vi "links weiter.vi"(8 "error in (no error)":errorcluster caption="Fehler (Eingang, kein Fehler)", 11 "Device ID":T1(ring)) -> (0 "error out":errorcluster caption="Fehler (Ausgang)", 2 "geradeaus?":bool, 3 "Device ID Out":T1(ring))   [LabVIEW 2010]
uses:
  globale Variable 1.vi
panel:
  out "aktuelle Position":i32
  in  "pneumatik?":bool
  in  "ende?":bool
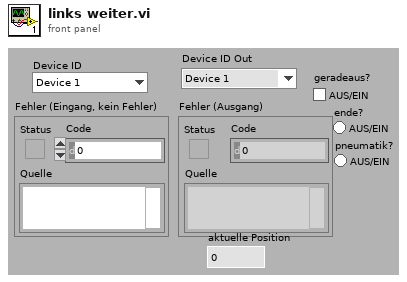
[diagram p1: front panel]
types:
  T1 = enum16{"Device 1", "Device 2", "Device 3", "Device 4", "Device 5", "Device 6", "Device 7", "Device 8"}
  T2 = enum8{"Output 1 (O1)", "Output 2 (O2)", "Output 3 (O3)", "Output 4 (O4)", "Output 5 (O5)", "Output 6 (O6)", "Output 7 (O7)", "Output 8 (O8)"}
  T3 = enum8{"Robo Interface", "Extension 1", "Extension 2", "Extension 3"}
  T4 = enum8{"Power 1", "Power 2", "Power 3", "Power 4", "Power 5", "Power 6", "Power 7", "Power 8"}
  T5 = enum8{"Input 1 (I1)", "Input 2 (I2)", "Input 3 (I3)", "Input 4 (I4)", "Input 5 (I5)", "Input 6 (I6)", "Input 7 (I7)", "Input 8 (I8)"}
  T6 = enum8{"Goes High", "Goes Low", "Goes High or Low"}
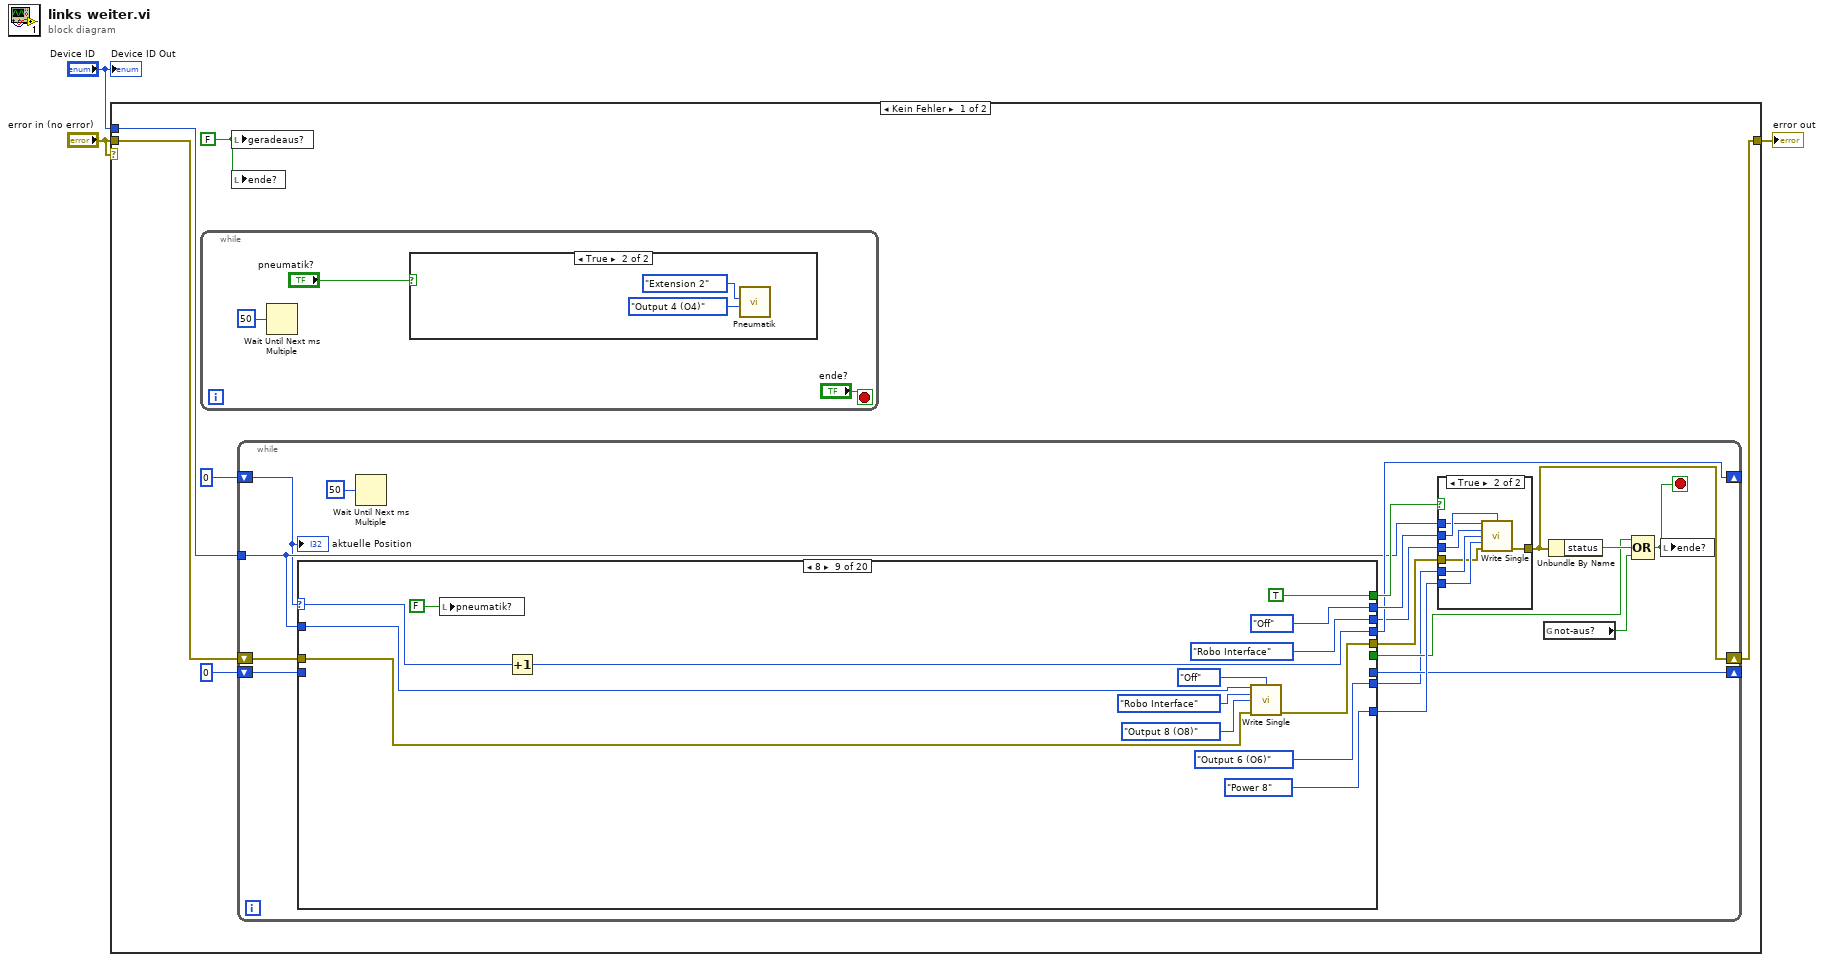
[diagram p0: block diagram]
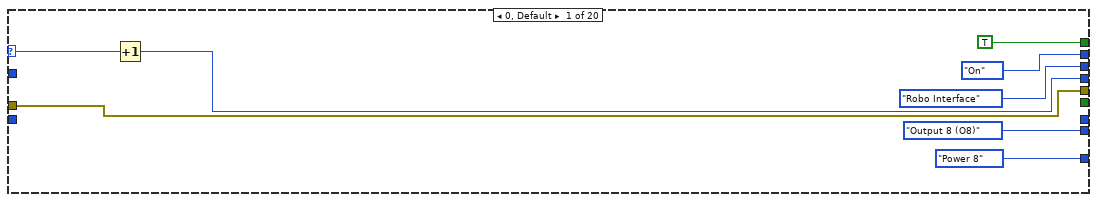
[diagram p3: hidden frame]
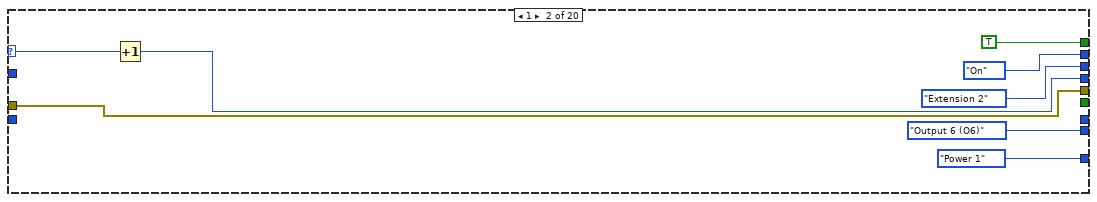
[diagram p4: hidden frame]
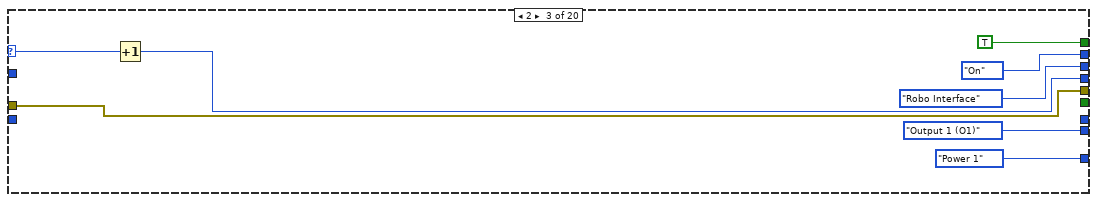
[diagram p5: hidden frame]
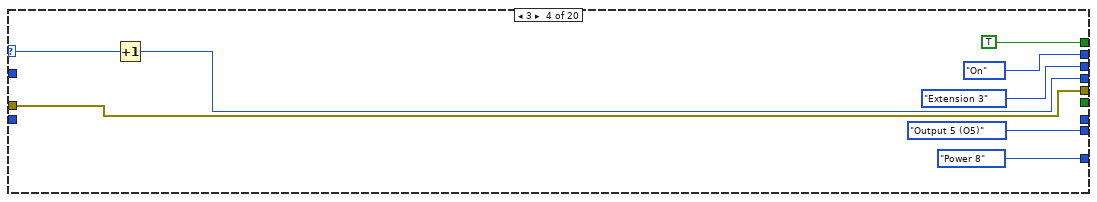
[diagram p6: hidden frame]
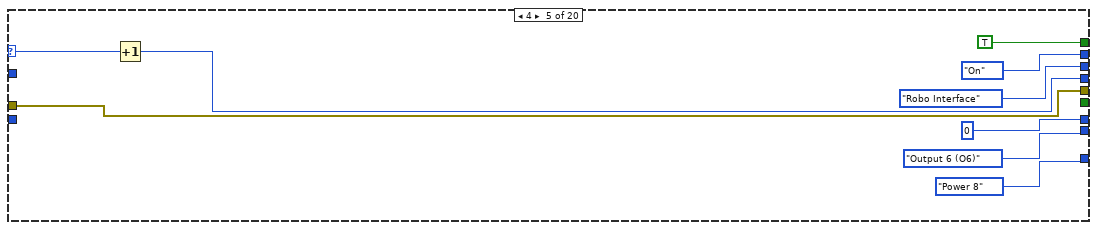
[diagram p7: hidden frame]
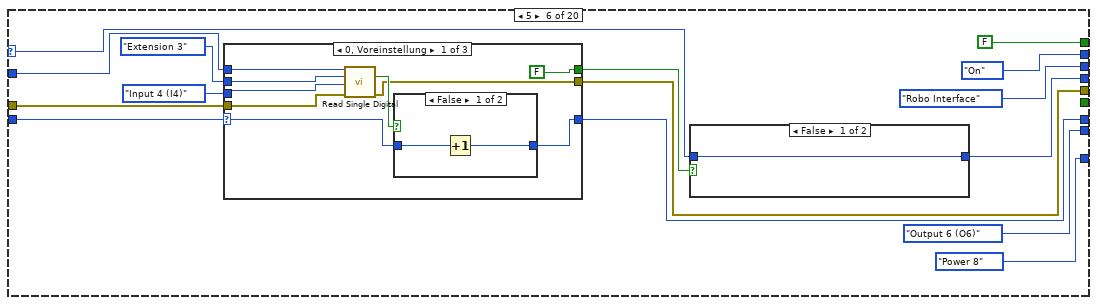
[diagram p8: hidden frame]
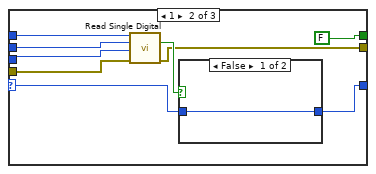
[diagram p10: hidden frame]
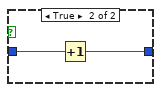
[diagram p11: hidden frame]
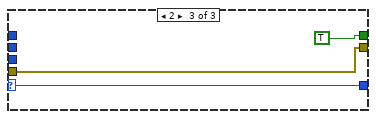
[diagram p12: hidden frame]
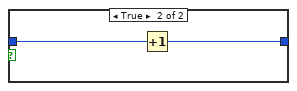
[diagram p13: hidden frame]
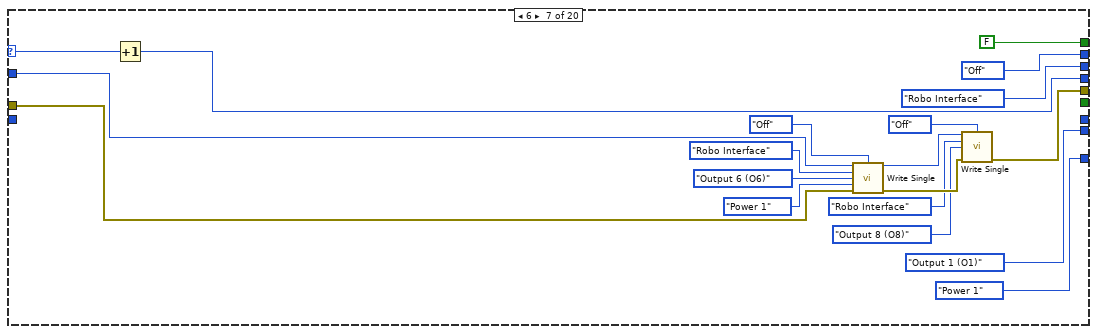
[diagram p14: hidden frame]
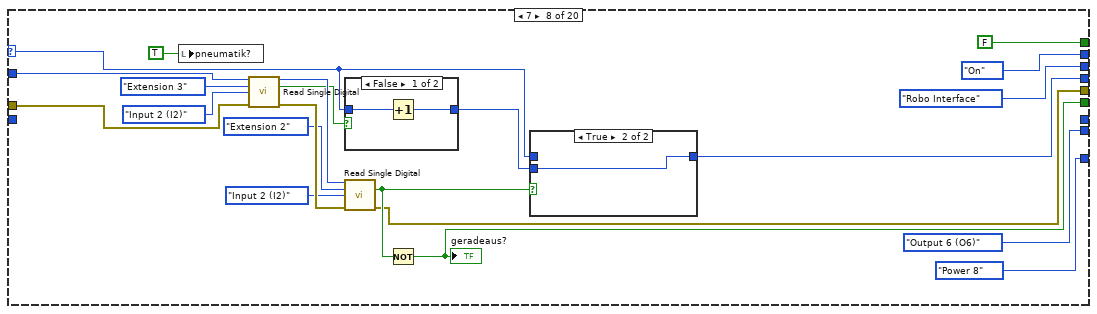
[diagram p15: hidden frame]
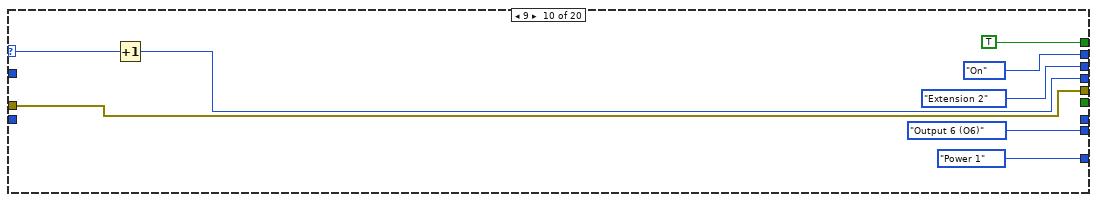
[diagram p18: hidden frame]
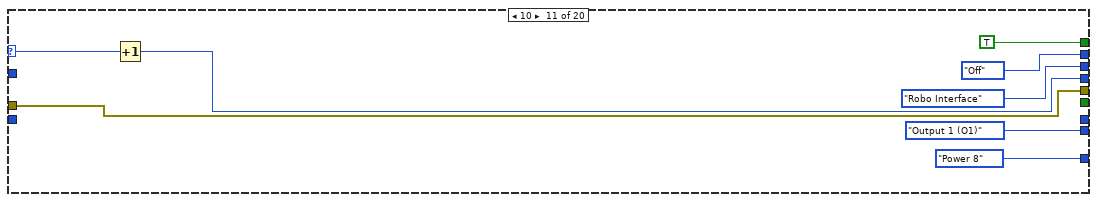
[diagram p19: hidden frame]
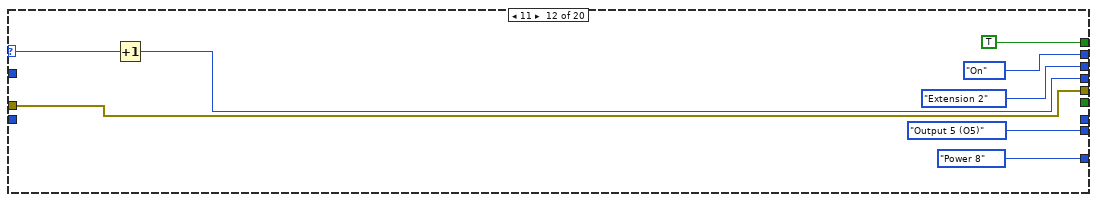
[diagram p20: hidden frame]
diagram:
  n1 = case shown="Kein Fehler" "error in (no error)" {
    tunnel: "Device ID" -> [w8 _]
    tunnel: [w7 w293] -> w3
    tunnel: "error in (no error)" -> [w6 w293]
    frame No Error {
      w4 = FALSE ("geradeaus?")
      n2 = while {
        stop <- "ende?" stop-if-true
        n3 = Wait Until Next ms Multiple(millisecond multiple=50) -> ()  [unwired: 1 out]
        n4 = case shown="True" "pneumatik?" {
          frame False {
          }
          frame True {
            n5 = call "Pneumatik.vi"("Single_Output"=T2."Output 4 (O4)", "Module"=T3."Extension 2") -> ()  [unwired: 2 in, 8 out]
          }
        }
      }
      n6 = local write "geradeaus?"(w4) -> ()
      n7 = local write "ende?"(w4) -> ()
      n8 = while {
        shift-right: [w27] -> _
        shift-left: 0 -> [w15]
        tunnel: w8 -> [w16]
        shift-right: [w25] -> w7
        shift-left: w6 -> [w29]
        shift-right: [w21] -> _
        shift-left: 0 -> [w22]
        stop <- w19 stop-if-true
        n9 = case shown="8" w15 {
          selector: w15 -> [w34 w42 w50 w58 w68 w83 w131 w143 w171 w179 w187 w195 w203 w224 w231 w244 w252 w261 w270 w279]
          tunnel: [TRUE ("AN/Aus") TRUE ("AN/Aus") TRUE ("AN/Aus") TRUE ("AN/Aus") TRUE ("AN/Aus") FALSE ("AN/Aus") FALSE ("AN/Aus") FALSE ("AN/Aus") TRUE ("AN/Aus") TRUE ("AN/Aus") TRUE ("AN/Aus") TRUE ("AN/Aus") TRUE ("AN/Aus") FALSE ("AN/Aus") TRUE ("AN/Aus") FALSE ("AN/Aus") TRUE ("AN/Aus") FALSE ("AN/Aus") TRUE ("AN/Aus") FALSE ("AN/Aus")] -> w32
          tunnel: [enum8{"Off", "On"}."On" ("Output_Action") enum8{"Off", "On"}."On" ("Output_Action") enum8{"Off", "On"}."On" ("Output_Action") enum8{"Off", "On"}."On" ("Output_Action") enum8{"Off", "On"}."On" ("Output_Action") enum8{"Off", "On"}."On" ("Output_Action") enum8{"Off", "On"}."Off" ("Output_Action") enum8{"Off", "On"}."On" ("Output_Action") enum8{"Off", "On"}."Off" ("Output_Action") enum8{"Off", "On"}."On" ("Output_Action") enum8{"Off", "On"}."Off" ("Output_Action") enum8{"Off", "On"}."On" ("Output_Action") enum8{"Off", "On"}."Off" ("Output_Action") enum8{"Off", "On"}."Off" ("Output_Action") enum8{"Off", "On"}."Off" ("Output_Action") enum8{"Off", "On"}."Off" ("Output_Action") enum8{"Off", "On"}."Off" ("Output_Action") enum8{"Off", "On"}."Off" ("Output_Action") enum8{"Off", "On"}."Off" ("Output_Action") enum8{"Off", "On"}."Off" ("Output_Action")] -> w31
          tunnel: [T2."Output 8 (O8)" ("Single_Output") T2."Output 6 (O6)" ("Single_Output") T2."Output 1 (O1)" ("Single_Output") T2."Output 5 (O5)" ("Single_Output") T2."Output 6 (O6)" ("Single_Output") T2."Output 6 (O6)" ("Single_Output") T2."Output 1 (O1)" ("Single_Output") T2."Output 6 (O6)" ("Single_Output") T2."Output 6 (O6)" ("Single_Output") T2."Output 6 (O6)" ("Single_Output") T2."Output 1 (O1)" ("Single_Output") T2."Output 5 (O5)" ("Single_Output") T2."Output 5 (O5)" ("Single_Output") T2."Output 1 (O1)" ("Single_Output") T2."Output 6 (O6)" ("Single_Output") T2."Output 6 (O6)" ("Single_Output") T2."Output 8 (O8)" ("Single_Output") T2."Output 6 (O6)" ("Single_Output") T2."Output 5 (O5)" ("Single_Output") T2."Output 5 (O5)" ("Single_Output")] -> w17
          tunnel: [T4."Power 8" ("Output_PWM") T4."Power 1" ("Output_PWM") T4."Power 1" ("Output_PWM") T4."Power 8" ("Output_PWM") T4."Power 8" ("Output_PWM") T4."Power 8" ("Output_PWM") T4."Power 1" ("Output_PWM") T4."Power 8" ("Output_PWM") T4."Power 8" ("Output_PWM") T4."Power 1" ("Output_PWM") T4."Power 8" ("Output_PWM") T4."Power 8" ("Output_PWM") T4."Power 8" ("Output_PWM") T4."Power 8" ("Output_PWM") T4."Power 8" ("Output_PWM") T4."Power 8" ("Output_PWM") T4."Power 8" ("Output_PWM") T4."Power 8" ("Output_PWM") T4."Power 8" ("Output_PWM") T4."Power 8" ("Output_PWM")] -> w30
          tunnel: [T3."Robo Interface" ("Module") T3."Extension 2" ("Module") T3."Robo Interface" ("Module") T3."Extension 3" ("Module") T3."Robo Interface" ("Module") T3."Robo Interface" ("Module") T3."Robo Interface" ("Module") T3."Robo Interface" ("Module") T3."Robo Interface" ("Module") T3."Extension 2" ("Module") T3."Robo Interface" ("Module") T3."Extension 2" ("Module") T3."Extension 3" ("Module") T3."Robo Interface" ("Module") T3."Extension 2" ("Module") T3."Extension 2" ("Module") T3."Robo Interface" ("Module") T3."Extension 2" ("Module") T3."Extension 2" ("Module") T3."Extension 2" ("Module")] -> w18
          tunnel: w16 -> [_ _ _ _ _ w81 w126 w145 w166 _ _ _ _ w223 _ w243 _ _ _ _]
          tunnel: w29 -> [w35 w43 w51 w59 w65 w74 w125 w144 w165 w178 w186 w194 w202 w222 w232 w242 w251 w260 w269 w278]
          tunnel: [w35 w43 w51 w59 w65 w80 w122 w140 w164 w178 w186 w194 w202 w217 w232 w241 w251 w260 w269 w278] -> w28
          tunnel: [w33 w41 w49 w57 w67 w82 w132 w147 w172 w180 w188 w196 w204 w225 w233 w245 w253 w259 w267 w276] -> w27
          tunnel: w22 -> [_ _ _ _ _ w78 _ _ _ _ _ _ _ _ _ _ _ _ _ _]
          tunnel: [_ _ _ _ 0 w75 _ _ _ _ _ _ _ _ _ _ _ _ _ _] -> w21
          tunnel: [_ _ _ _ _ _ _ w138 _ _ _ _ _ _ _ _ _ _ FALSE TRUE] -> w20
          frame 0, Default {
            n10 = Increment(x=w34) -> (x+1=w33:i32)
          }
          frame 1 {
            n11 = Increment(x=w42) -> (x+1=w41:i32)
          }
          frame 2 {
            n12 = Increment(x=w50) -> (x+1=w49:i32)
          }
          frame 3 {
            n13 = Increment(x=w58) -> (x+1=w57:i32)
          }
          frame 4 {
            n14 = Increment(x=w68) -> (x+1=w67:i32)
          }
          frame 5 {
            n15 = case shown="0, Voreinstellung" w78 {
              selector: w78 -> [w96 w108 w114]
              tunnel: w81 -> [w92 w103 _]
              tunnel: w74 -> [w91 w104 w113]
              tunnel: [w89 w101 w113] -> w80
              tunnel: [FALSE ("Value") FALSE ("Value") TRUE ("Value")] -> w79
              tunnel: T3."Extension 3" ("Module") -> [w93 w106 _]
              tunnel: T5."Input 4 (I4)" ("Digital_Input") -> [w94 w105 _]
              tunnel: [w95 w107 w114] -> w75
              frame 0, Default {
                n16 = call "Read Single Digital.vi"("Device ID"=w92, "Module"=w93, "Digital_Input"=w94, "error in"=w91) -> ("Value"=w90:bool, "error out"=w89:errorcluster)  [unwired: 10 out]
                n17 = case shown="False" w90 {
                  tunnel: w96 -> [w99 w100]
                  tunnel: [w98 w100] -> w95
                  frame False {
                    n18 = Increment(x=w99) -> (x+1=w98:i32)
                  }
                  frame True {
                  }
                }
              }
              frame 1 {
                n19 = call "Read Single Digital.vi"("Device ID"=w103, "Module"=w106, "Digital_Input"=w105, "error in"=w104) -> ("Value"=w102:bool, "error out"=w101:errorcluster)  [unwired: 10 out]
                n20 = case shown="False" w102 {
                  tunnel: w108 -> [w110 w112]
                  tunnel: [w110 w111] -> w107
                  frame False {
                  }
                  frame True {
                    n21 = Increment(x=w112) -> (x+1=w111:i32)
                  }
                }
              }
              frame 2 {
              }
            }
            n22 = case shown="False" w79 {
              tunnel: w83 -> [w116 w118]
              tunnel: [w116 w117] -> w82
              frame False {
              }
              frame True {
                n23 = Increment(x=w118) -> (x+1=w117:i32)
              }
            }
          }
          frame 6 {
            n24 = Increment(x=w131) -> (x+1=w132:i32)
            n25 = call "Write Single.vi"("Device ID"=w126, "Output_Action"=enum8{"Off", "On"}."Off", "Module"=T3."Robo Interface", "Single_Output"=T2."Output 6 (O6)", "Output_PWM"=T4."Power 1", "error in"=w125) -> ("Device ID Out"=w124:T1, "error out"=w123:errorcluster)  [unwired: 8 out]
            n26 = call "Write Single.vi"("Device ID"=w124, "Output_Action"=enum8{"Off", "On"}."Off", "Module"=T3."Robo Interface", "Single_Output"=T2."Output 8 (O8)", "error in"=w123) -> ("error out"=w122:errorcluster)  [unwired: 1 in, 9 out]
          }
          frame 7 {
            n27 = local write "pneumatik?"(TRUE ("pneumatik?")) -> ()
            n28 = call "Read Single Digital.vi"("Device ID"=w145, "Module"=T3."Extension 3", "Digital_Input"=T5."Input 2 (I2)", "error in"=w144) -> ("Device ID Out"=w152:T1, "Value"=w146:bool, "error out"=w151:errorcluster)  [unwired: 9 out]
            n29 = case shown="False" w146 {
              tunnel: w143 -> [w160 w161]
              tunnel: [w159 w161] -> w148
              frame False {
                n30 = Increment(x=w160) -> (x+1=w159:i32)
              }
              frame True {
              }
            }
            n31 = call "Read Single Digital.vi"("Device ID"=w152, "Module"=T3."Extension 2", "Digital_Input"=T5."Input 2 (I2)", "error in"=w151) -> ("Value"=w142:bool, "error out"=w140:errorcluster)  [unwired: 10 out]
            n32 = Not(x=w142) -> (.not. x?=w138:bool)
            "geradeaus?" <- w138
            n33 = case shown="True" w142 {
              tunnel: w148 -> [_ w163]
              tunnel: [w162 w163] -> w147
              tunnel: w143 -> [w162 _]
              frame False {
              }
              frame True {
              }
            }
          }
          frame 8 {
            n34 = local write "pneumatik?"(FALSE ("pneumatik?")) -> ()
            n35 = Increment(x=w171) -> (x+1=w172:i32)
            n36 = call "Write Single.vi"("Device ID"=w166, "Output_Action"=enum8{"Off", "On"}."Off", "Module"=T3."Robo Interface", "Single_Output"=T2."Output 8 (O8)", "error in"=w165) -> ("error out"=w164:errorcluster)  [unwired: 1 in, 9 out]
          }
          frame 9 {
            n37 = Increment(x=w179) -> (x+1=w180:i32)
          }
          frame 10 {
            n38 = Increment(x=w187) -> (x+1=w188:i32)
          }
          frame 11 {
            n39 = Increment(x=w195) -> (x+1=w196:i32)
          }
          frame 12 {
            n40 = Increment(x=w203) -> (x+1=w204:i32)
          }
          frame 13 {
            n41 = Increment(x=w224) -> (x+1=w225:i32)
            n42 = call "Wait Until Digital Edge.vi"("Device ID"=w223, "Wait Until"=T6."Goes High", "Module"=T3."Extension 2", "Digital_Input"=T5."Input 6 (I6)", "error in"=w222, "Time Out (10)"=inf) -> ("Device ID Out"=w210:T1, "error out"=w212:errorcluster)  [unwired: 8 out]
            n43 = call "Write Single.vi"("Device ID"=w210, "Output_Action"=enum8{"Off", "On"}."On", "Module"=T3."Robo Interface", "Single_Output"=T2."Output 8 (O8)", "Output_PWM"=T4."Power 8", "error in"=w212) -> ("error out"=w211:errorcluster)  [unwired: 9 out]
            n44 = call "Verzögerung"("error in (no error)"=w211) -> ("error out"=w217:errorcluster)  [unwired: 1 in, 9 out]
          }
          frame 14 {
            n45 = Increment(x=w231) -> (x+1=w233:i32)
          }
          frame 15 {
            n46 = Increment(x=w244) -> (x+1=w245:i32)
            n47 = call "Pneumatik.vi"("error in (no error)"=w242, "Single_Output"=T2."Output 1 (O1)", "Module"=T3."Extension 2", "Device ID"=w243) -> ("error out"=w241:errorcluster)  [unwired: 7 out]
          }
          frame 16 {
            n48 = Increment(x=w252) -> (x+1=w253:i32)
          }
          frame 17 {
            n49 = Increment(x=w261) -> (x+1=w259:i32)
          }
          frame 18 {
            n50 = Increment(x=w270) -> (x+1=w267:i32)
          }
          frame 19 {
            n51 = Increment(x=w279) -> (x+1=w276:i32)
          }
        }
        n52 = Wait Until Next ms Multiple(millisecond multiple=50) -> ()  [unwired: 1 out]
        n53 = case shown="True" w32 {
          tunnel: [w285 w292] -> w25
          tunnel: w31 -> [_ w291]
          tunnel: w17 -> [_ w290]
          tunnel: w30 -> [_ w289]
          tunnel: w18 -> [_ w288]
          tunnel: w16 -> [_ w287]
          tunnel: w28 -> [w285 w286]
          frame False {
          }
          frame True {
            n54 = call "Write Single.vi"("Device ID"=w287, "Output_Action"=w291, "Module"=w288, "Single_Output"=w290, "Output_PWM"=w289, "error in"=w286) -> ("error out"=w292:errorcluster)  [unwired: 9 out]
          }
        }
        n55 = global read "globale Variable 1.vi" "not-aus?"() -> (w23:bool)
        n56 = Unbundle By Name(w25) -> ("status"=w24:bool)
        n57 = Compound Arithmetic op=OR(w20, w24, w23) -> (w19:bool)
        n58 = local write "ende?"(w19) -> ()
        "aktuelle Position" <- w15
      }
    }
    frame Error {
    }
  }
  "error out" <- w3
  "Device ID Out" <- "Device ID"
